vi "set mappings by module.vi"(8 "error in":errorcluster, 9 "module mappings":T1, 10 "owner ID":string, 11 "engine configuration in":refnum<class "engine configuration.lvclass">) -> (0 "error out":errorcluster, 3 "engine configuration out":refnum<class "engine configuration.lvclass">)   [LabVIEW 2013, in "engine configuration.lvclass"]
uses:
  engine configuration.lvclass
  Module Mappings.ctl
  <vilib>/NI/Tag Bus/table/mapping specification.ctl
  <vilib>/NI/Tag Bus/tag/Data Type.ctl
  <vilib>/NI/Tag Bus/table/mapping.ctl
  engine configuration.lvclass/engine configuration.ctl
  <vilib>/NI/Tag Bus/table/data table.lvlib
  <vilib>/NI/Tag Bus/tag/tag descriptor.lvclass
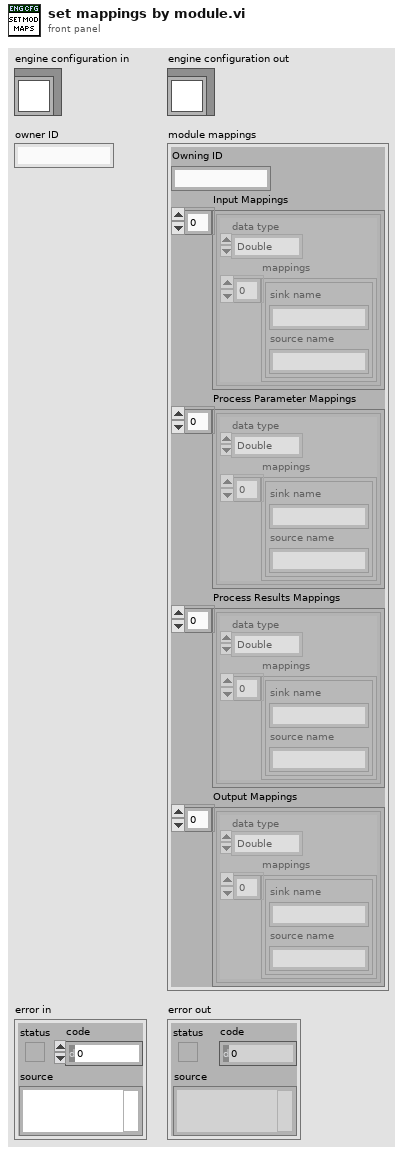
[diagram p1: front panel]
types:
  T1 = typedef "engine configuration.lvclass/Module Mappings.ctl" = cluster{"Owning ID":string, "Input Mappings":T2[], "Process Parameter Mappings":T2[], "Process Results Mappings":T2[], "Output Mappings":T2[]}
  T2 = typedef "tag bus.lvlib/data table.lvlib/mapping specification.ctl" = cluster{"data type":T3, "mappings":T4[]}
  T3 = typedef "tag bus.lvlib/tag descriptor.lvclass/Data Type.ctl" = enum16{"Double", "Single", "I64", "I32", "I16", "I8", "U64", "U32", "U16", "U8", "Boolean", "String", "Array of Double", "Array of Single", "Array of I64", "Array of I32", "Array of I16", "Array of I8", "Array of U64", "Array of U32", "Array of U16", "Array of U8", "Array of Boolean", "Array of String"}
  T4 = typedef "tag bus.lvlib/data table.lvlib/mapping.ctl" = cluster{"sink name":string, "source name":string}
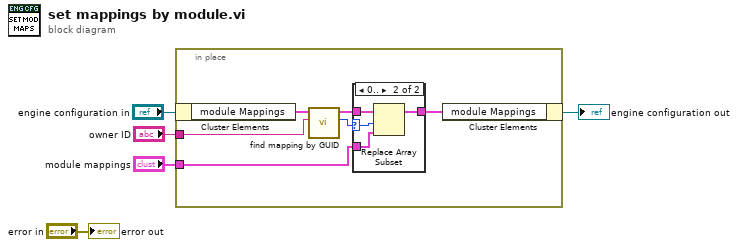
[diagram p0: block diagram]
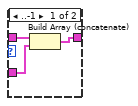
[diagram p2: hidden frame]
diagram:
  n1 = in-place {
    in-place-border: "owner ID" -> [w10]
    in-place-border: "module mappings" -> [w7]
    n2 = in-place-cluster #1("engine configuration in") -> ("module Mappings"=w11:T1[])
    n3 = call "find mapping by GUID.vi"("owner ID"=w10, "module Mappings"=w11) -> ("index"=w9:i32, "module Mappings out"=w8:T1[])  [unwired: 8 in]
    n4 = case shown="0.." w9 {
      selector: w9 -> [_ w17]
      tunnel: w8 -> [w13 w18]
      tunnel: w7 -> [w14 w16]
      tunnel: [w12 w15] -> w6
      frame ..-1 {
        n5 = Build Array (concatenate)(w13, w14) -> (w12:T1[])
      }
      frame 0.. {
        n6 = Replace Array Subset(array=w18, new element=w16, index=w17) -> (w15:T1[])
      }
    }
    n7 = in-place-cluster #1("module Mappings"=w6) -> (→"engine configuration out":refnum<class "engine configuration.lvclass">)
  }
  "error out" <- "error in"
